vi "Pre Launch Init.vi"(11 "State Machine in":refnum<class "State Machine.lvclass">) -> (0 "error out":errorcluster, 3 "State Machine out":refnum<class "State Machine.lvclass">)   [LabVIEW 2024, in "State Machine.lvlib" / "State Machine.lvclass"]
doc: "<p>(<strong>Filename</strong>: <span class=\"dnl\">Actor Framework.lvlib:Actor.lvclass:Pre Launch Init.vi</span>)</p>\n<p>Defines behavior that occurs after the <a href=\"nihelplauncher://docs/csh?context=lvcore_lvcomm_af_launch_nested_actor\">Launch Nested Actor</a> method is invoked but before the actor's Actor Core method begins running.</p>\n<p>By default, this method does nothing. A descendant class may override it to define behavior.</p>"
uses:
  State Machine.lvclass
  State/Idle/Idle.lvclass
  C:/Users/uspoaotto/OneDrive - Oregon Tool/Desktop/temp/actor framework state machine/State Machine/State/State/State.lvclass
  State Machine.lvclass/State Machine.ctl
  <vilib>/ActorFramework/Actor/Actor.lvclass
  Context/Context/Context.lvclass
  C:/Program Files (x86)/National Instruments/LabVIEW 2024/vi.lib/ActorFramework/Actor/Actor.lvclass
  C:/Users/uspoaotto/OneDrive - Oregon Tool/Desktop/temp/actor framework state machine/State Machine/State Machine/State Machine.lvclass
  C:/Users/uspoaotto/OneDrive - Oregon Tool/Desktop/temp/actor framework state machine/State Machine/State/Idle/Idle.lvclass
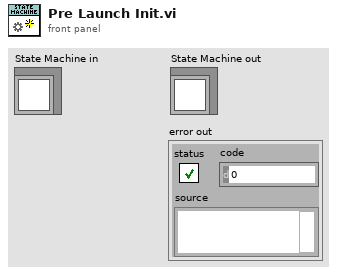
[diagram p1: front panel]
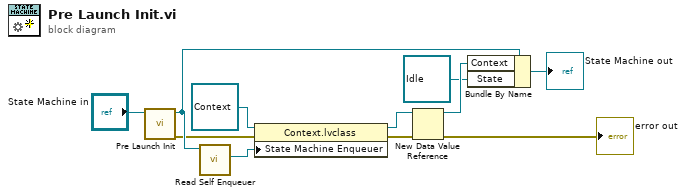
[diagram p0: block diagram]
diagram:
  n1 = call-parent "Pre Launch Init.vi"("Actor in"="State Machine in") -> ("error out"=w3:errorcluster, "Actor out"=w6:refnum<class "State Machine.lvclass">)  [unwired: 9 in]
  n2 = call <vilib>:"Read Self Enqueuer.vi"("Actor"=w6) -> ("Self Enqueuer"=w4:refnum<class "Message Enqueuer.lvclass">)  [unwired: 10 in]
  n3 = property class="Context.lvclass"(reference=refnum<class "Context.lvclass"> refnum ("Context.lvlib:Context.lvclass"), error in=w3, "State Machine Enqueuer"=w4) -> (reference out=w1:refnum<class "Context.lvclass">, error out=w2:errorcluster)
  n4 = New Data Value Reference(data value=w1, error in=w2) -> (data value reference=w10:refnum<data-value>, error out=→"error out":errorcluster)
  n5 = Bundle By Name(cluster=w6, "Context"=w10, "State"=refnum<class "Idle.lvclass"> refnum ("State.lvlib:Idle.lvclass")) -> (→"State Machine out":refnum<class "State Machine.lvclass">)
